vi "On Failure.vi"(8 "error in (no error)":errorcluster, 9 "Session In":refnum<class "Session.lvclass">, 11 "FormAuthentication in":refnum<class "FormAuthentication.lvclass">) -> (0 "error out":errorcluster, 1 "Session":refnum<class "Session.lvclass">, 2 "Response":refnum<class "Response.lvclass">, 3 "FormAuthentication out":refnum<class "FormAuthentication.lvclass">)   [LabVIEW 2020, in "HTTP Server.lvlib" / "FormAuthentication.lvclass"]
uses:
  FormAuthentication.lvclass
  <vilib>/IlluminatedG/IG HTTP Utils/HTTP Utils/Response/Response.lvclass
  FormAuthentication.lvclass/FormAuthentication.ctl
  Session/Session.lvclass
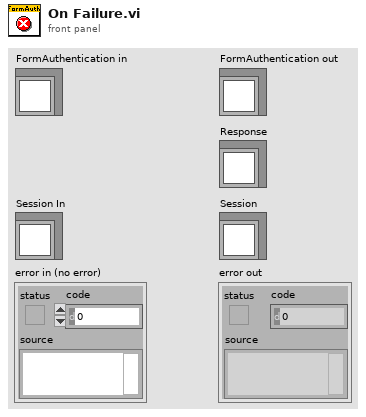
[diagram p1: front panel]
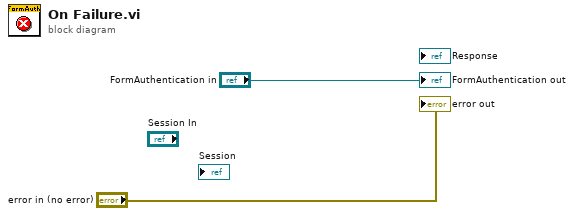
[diagram p0: block diagram]
diagram:
  "error out" <- "error in (no error)"
  "FormAuthentication out" <- "FormAuthentication in"
